vi "NISE.local.Rename Device.vi"(0 "SLSC Local in":refnum<class "SLSC Interface.lvclass">, 5 "device":refnum<k21>, 7 "new device name":string, 11 "error in (no error)":errorcluster) -> (4 "SLSC Local out":refnum<class "SLSC Interface.lvclass">, 15 "error out":errorcluster)   [LabVIEW 2016, in "SLSC Interface.lvclass"]
uses:
  SLSC Interface Class/SLSC Interface.lvclass
  SLSC Interface Class/NISE.Read session.vi
  SLSC Interface Class/NISE.Write session.vi
  <vilib>/SLSC/SLSC.lvlib
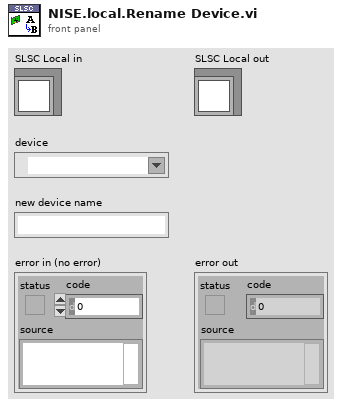
[diagram p1: front panel]
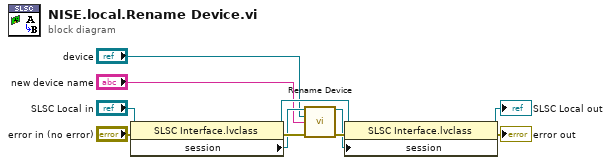
[diagram p0: block diagram]
diagram:
  n1 = property class="SLSC Interface.lvclass"(reference="SLSC Local in", error in="error in (no error)") -> (reference out=w9:refnum<class "SLSC Interface.lvclass">, error out=w11:errorcluster, "session"=w8:refnum<k21>)
  n2 = call <vilib>:"Rename Device.vi"("session in"=w8, "device"="device", "new device name"="new device name", "error in (no error)"=w11) -> ("session out"=w7:refnum<k21>, "error out"=w10:errorcluster)  [unwired: 10 in]
  n3 = property class="SLSC Interface.lvclass"(reference=w9, error in=w10, "session"=w7) -> (reference out=→"SLSC Local out":refnum<class "SLSC Interface.lvclass">, error out=→"error out":errorcluster)
